vi "Create Indices.vi"(0 "Component Mappings":T7, 5 "main data dictionary":refnum<class "data dictionary.lvclass">, 7 "data description":T5, 11 "error in":errorcluster) -> (4 "Input Transfer Specification":T1, 6 "Parameter Transfer Specifcation":T1, 8 "Result Transfer Specifcation":T1, 10 "Output Transfer Specifcation":T1, 15 "error out":errorcluster)   [LabVIEW 2013, in "Standard Engine Runtime.lvclass"]
uses:
  Standard Engine Runtime.lvclass
  <vilib>/NI/Module Execution Interface/Engine Configuration/Module Mappings.ctl
  <vilib>/NI/Tag Bus/table/mapping specification.ctl
  <vilib>/NI/Tag Bus/tag/Data Type.ctl
  <vilib>/NI/Tag Bus/table/mapping.ctl
  <vilib>/NI/Tag Bus/dictionary/data dictionary.lvclass
  <vilib>/NI/Tag Bus Module Framework/channel/data tables.ctl
  <vilib>/NI/Tag Bus/dictionary table pair.ctl
  <vilib>/NI/Tag Bus/table/data table.ctl
  Data Table with Transfer Spec.ctl
  <vilib>/NI/Tag Bus/table/transfer specification.ctl
  <vilib>/NI/Tag Bus/tag/tag descriptor.lvclass
  <vilib>/NI/Tag Bus/table/data table.lvlib
  <vilib>/NI/Tag Bus Module Framework/channel/TBM channel.lvclass
  <vilib>/NI/Tag Bus/tag bus.lvlib
  <vilib>/NI/Module Execution Interface/Engine Configuration/engine configuration.lvclass
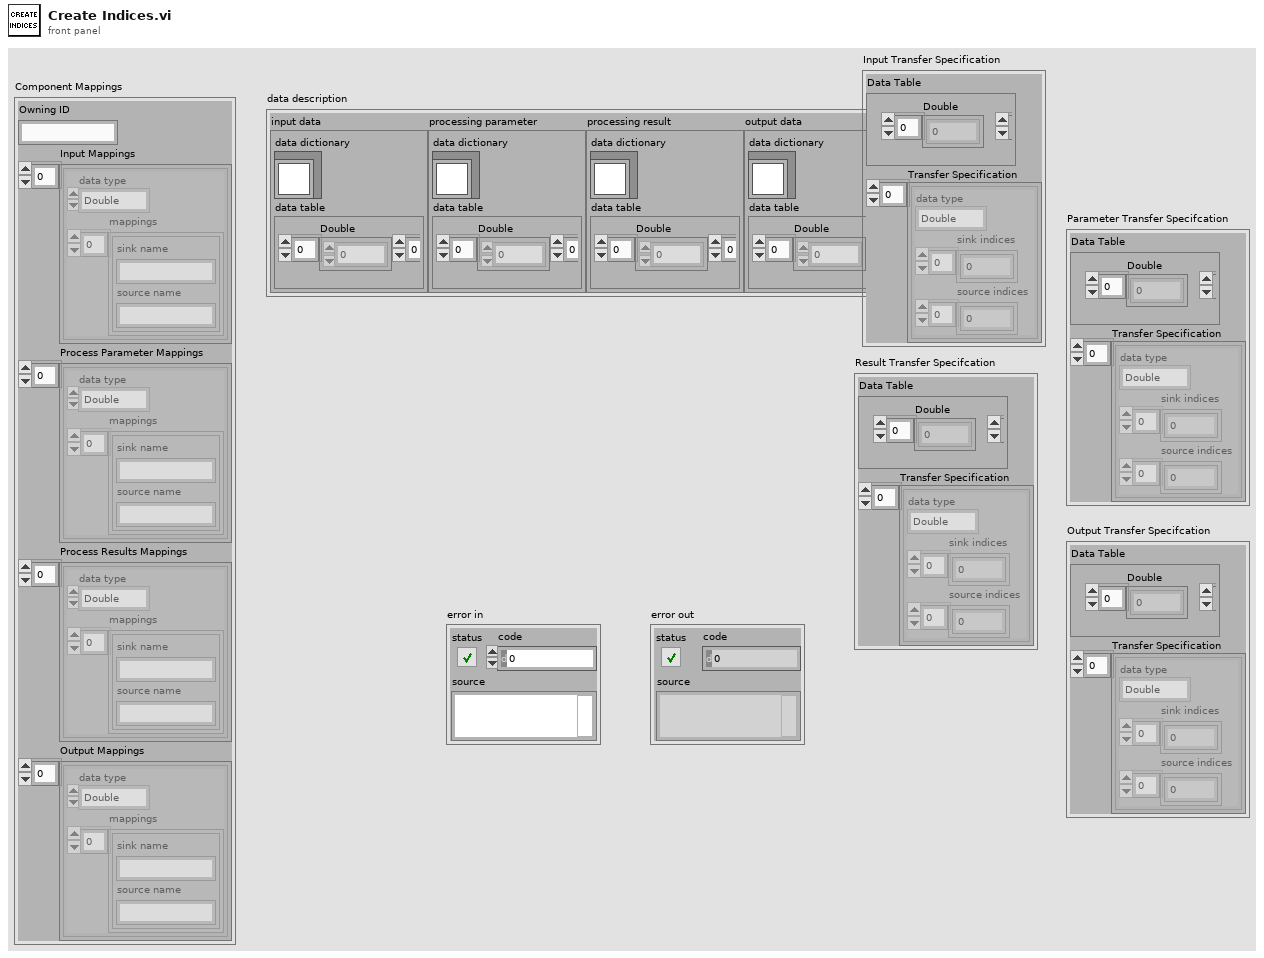
[diagram p1: front panel]
types:
  T1 = typedef "Standard Engine Runtime.lvclass/Data Table with Transfer Spec.ctl" = cluster{"Data Table":T2, "Transfer Specification":T3[]}
  T2 = typedef "tag bus.lvlib/data table.lvlib/data table.ctl" = cluster{"Double":dbl[], "Single":sgl[], "I64":i64[], "I32":i32[], "I16":i16[], "I8":i8[], "U64":u64[], "U32":u32[], "U16":u16[], "U8":u8[], "Boolean":bool[], "String":string[], "Array of Double":cluster{"DBL Array":dbl[]}[], "Array of Single":cluster{"SGL Array":sgl[]}[], "Array of I64":cluster{"I64 Array":i64[]}[], "Array of I32":cluster{"I32 Array":i32[]}[], "Array of I16":cluster{"I16 Array":i16[]}[], "Array of I8":cluster{"I8 Array":i8[]}[], "Array of U64":cluster{"U64 Array":u64[]}[], "Array of U32":cluster{"U32 Array":u32[]}[], "Array of U16":cluster{"U16 Array":u16[]}[], "Array of U8":cluster{"U8 Array":u8[]}[], "Array of Boolean":cluster{"Boolean Array":bool[]}[], "Array of String":cluster{"String Array":string[]}[]}
  T3 = typedef "tag bus.lvlib/data table.lvlib/transfer specification.ctl" = cluster{"data type":T4, "sink indices":i32[], "source indices":i32[]}
  T4 = typedef "tag bus.lvlib/tag descriptor.lvclass/Data Type.ctl" = enum16{"Double", "Single", "I64", "I32", "I16", "I8", "U64", "U32", "U16", "U8", "Boolean", "String", "Array of Double", "Array of Single", "Array of I64", "Array of I32", "Array of I16", "Array of I8", "Array of U64", "Array of U32", "Array of U16", "Array of U8", "Array of Boolean", "Array of String"}
  T5 = typedef "TBM channel.lvclass/data tables.ctl" = cluster{"input data":T6, "processing parameter":T6, "processing result":T6, "output data":T6}
  T6 = typedef "tag bus.lvlib/dictionary table pair.ctl" = cluster{"data dictionary":refnum<class "data dictionary.lvclass">, "data table":T2}
  T7 = typedef "engine configuration.lvclass/Module Mappings.ctl" = cluster{"Owning ID":string, "Input Mappings":T8[], "Process Parameter Mappings":T8[], "Process Results Mappings":T8[], "Output Mappings":T8[]}
  T8 = typedef "tag bus.lvlib/data table.lvlib/mapping specification.ctl" = cluster{"data type":T4, "mappings":T9[]}
  T9 = typedef "tag bus.lvlib/data table.lvlib/mapping.ctl" = cluster{"sink name":string, "source name":string}
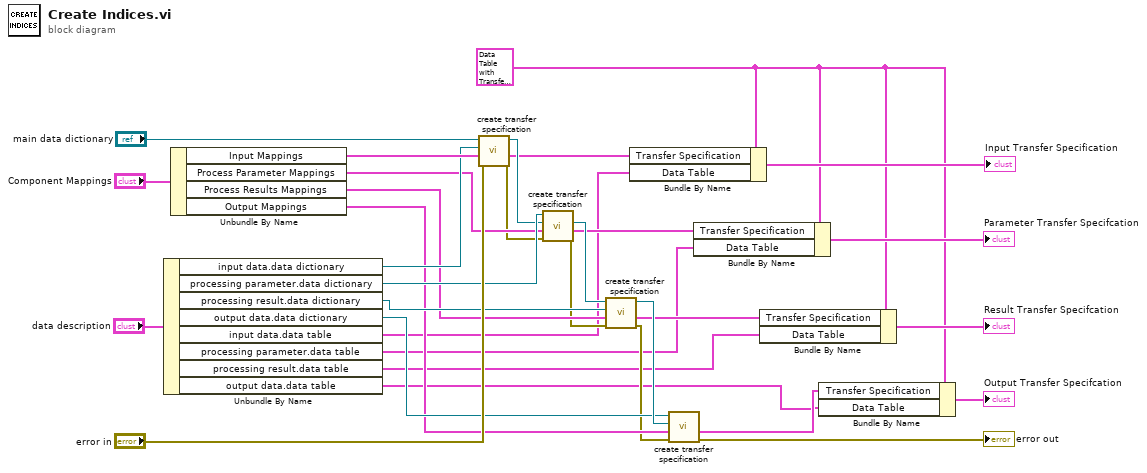
[diagram p0: block diagram]
diagram:
  w7 = T1 {"Data Table"={"Double"=[], "Single"=[], "I64"=[], "I32"=[], "I16"=[], "I8"=[], "U64"=[], "U32"=[], "U16"=[], "U8"=[], "Boolean"=[], "String"=[], "Array of Double"=[], "Array of Single"=[], "Array of I64"=[], "Array of I32"=[], "Array of I16"=[], "Array of I8"=[], "Array of U64"=[], "Array of U32"=[], "Array of U16"=[], "Array of U8"=[], "Array of Boolean"=[], "Array of String"=[]}, "Transfer Specification"=[]} ("Read Transfer Specification")
  n1 = Unbundle By Name("data description") -> ("input data.data dictionary"=w28:refnum<class "data dictionary.lvclass">, "processing parameter.data dictionary"=w26:refnum<class "data dictionary.lvclass">, "processing result.data dictionary"=w21:refnum<class "data dictionary.lvclass">, "output data.data dictionary"=w17:refnum<class "data dictionary.lvclass">, "input data.data table"=w4:T2, "processing parameter.data table"=w3:T2, "processing result.data table"=w2:T2, "output data.data table"=w1:T2)
  n2 = Unbundle By Name("Component Mappings") -> ("Input Mappings"=w29:T8[], "Process Parameter Mappings"=w24:T8[], "Process Results Mappings"=w20:T8[], "Output Mappings"=w16:T8[])
  n3 = call <vilib>:"create transfer specification.vi"("error in"="error in", "mapping specification"=w29, "data dictionary source in"=w28, "data dictionary sink in"="main data dictionary") -> ("error out"=w23:errorcluster, "transfer specification"=w13:T3[], "data dictionary sink out"=w25:refnum<class "data dictionary.lvclass">)  [unwired: 4 in, 1 out]
  n4 = call <vilib>:"create transfer specification.vi"("error in"=w23, "mapping specification"=w24, "data dictionary source in"=w25, "data dictionary sink in"=w26) -> ("error out"=w19:errorcluster, "transfer specification"=w11:T3[], "data dictionary source out"=w22:refnum<class "data dictionary.lvclass">)  [unwired: 4 in, 1 out]
  n5 = call <vilib>:"create transfer specification.vi"("error in"=w19, "mapping specification"=w20, "data dictionary source in"=w21, "data dictionary sink in"=w22) -> ("error out"=w15:errorcluster, "transfer specification"=w9:T3[], "data dictionary sink out"=w18:refnum<class "data dictionary.lvclass">)  [unwired: 4 in, 1 out]
  n6 = Bundle By Name(cluster=w7, "Transfer Specification"=w13, "Data Table"=w4) -> (→"Input Transfer Specification":T1)
  n7 = call <vilib>:"create transfer specification.vi"("error in"=w15, "mapping specification"=w16, "data dictionary source in"=w18, "data dictionary sink in"=w17) -> ("error out"=→"error out":errorcluster, "transfer specification"=w6:T3[])  [unwired: 4 in, 2 out]
  n8 = Bundle By Name(cluster=w7, "Transfer Specification"=w11, "Data Table"=w3) -> (→"Parameter Transfer Specifcation":T1)
  n9 = Bundle By Name(cluster=w7, "Transfer Specification"=w9, "Data Table"=w2) -> (→"Result Transfer Specifcation":T1)
  n10 = Bundle By Name(cluster=w7, "Transfer Specification"=w6, "Data Table"=w1) -> (→"Output Transfer Specifcation":T1)
